vi "InitVI UI.vi"() -> ()   [LabVIEW 2015, in "Initialization.lvclass"]
uses:
  Initialization.lvclass
  <vilib>/NI/Configuration Framework/Node/NodeRef.ctl
  <vilib>/NI/Configuration Framework/Node/NISE_CEF_Node.lvclass
  <vilib>/NI/AMC/Message Queue.ctl
  <vilib>/NI/AMC/Message.ctl
  <vilib>/NI/Tools/Keyed Array/KeyedArray.ctl
  <vilib>/NI/Configuration Framework/Node/UserEventRef.ctl
  <vilib>/NI/Configuration Framework/Controls/EventCluster.ctl
  XML Controls/Execution Types.ctl
  Initialization.lvclass/Initialization.ctl
  Read Initialization VI Properties.vi
  Write Initialization VI Properties.vi
  <vilib>/NI/AMC/Create Single Message.vi
  <vilib>/NI/AMC/Update Message Routing Info.vi
  <vilib>/NI/AMC/Send Message.vi
  <vilib>/NI/AMC/AMC.lvlib
  Configuration Tool.lvlib
  <vilib>/NI/Tools/Keyed Array/Tools_KeyedArray.lvlib
  <vilib>/NI/Configuration Framework/NISE_CEF_TreeControl.lvlib
  VeriStand Custom Device XML Parser.lvlib
panel:
  in  "Main UI Tab":enum32{"Initialization VI"}(tab)
  in  "Show Documentation":bool
  in  "Execution":T1
  in  "Type":enum16{"Action", "VI"}(ring)
  in  "Position":enum16{"centered", "mouse pointer"}(ring)
  in  "Host Path to Initialization VI":path
  in  "user event":T2
  in  "main queue":T3
  in  "node ref":T4
  # "Dialog Settings"
  # "Dialog Settings"
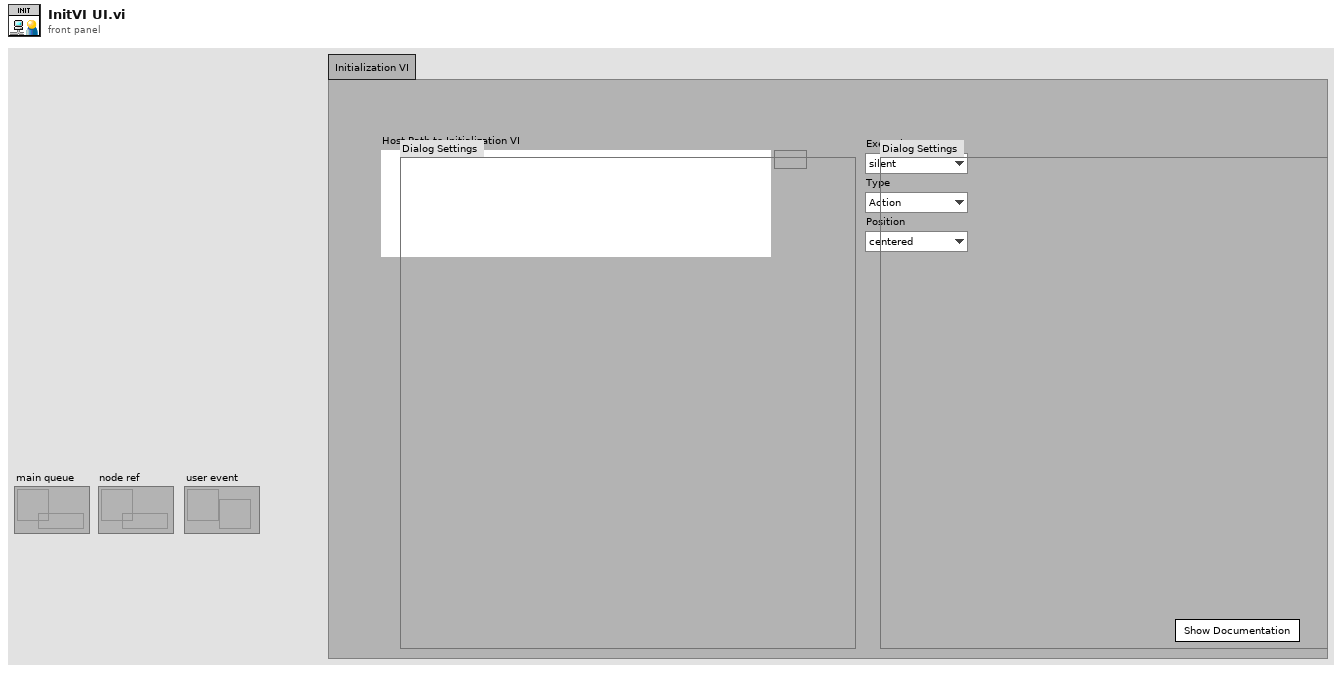
[diagram p1: front panel]
types:
  T1 = typedef "VeriStand Custom Device XML Parser.lvlib/Execution Types.ctl" = enum16{"silent", "modal", "floating", "default"}
  T2 = typedef "NISE_CEF_Node.lvclass/UserEventRef.ctl" = refnum<user-event>
  T3 = typedef "AMC.lvlib/Message Queue.ctl" = refnum<queue>
  T4 = typedef "NISE_CEF_Node.lvclass/NodeRef.ctl" = refnum<data-value>
  T5 = typedef "Initialization VI Properties.ctl" = cluster{"Execution":T6, "Path":T7, "Type":enum16{"Action", "VI"}, "Position":enum16{"centered", "mouse pointer"}}
  T6 = typedef "Execution Types.ctl" = enum16{"silent", "modal", "floating", "default"}
  T7 = typedef "Path Cluster.ctl" = cluster{"Path":path, "Path Type":enum16{"Absolute", "To Base", "To Common Doc Dir", "To Application Data Dir"}}
  T8 = enum16{"Absolute", "To Base", "To Common Doc Dir", "To Application Data Dir"}
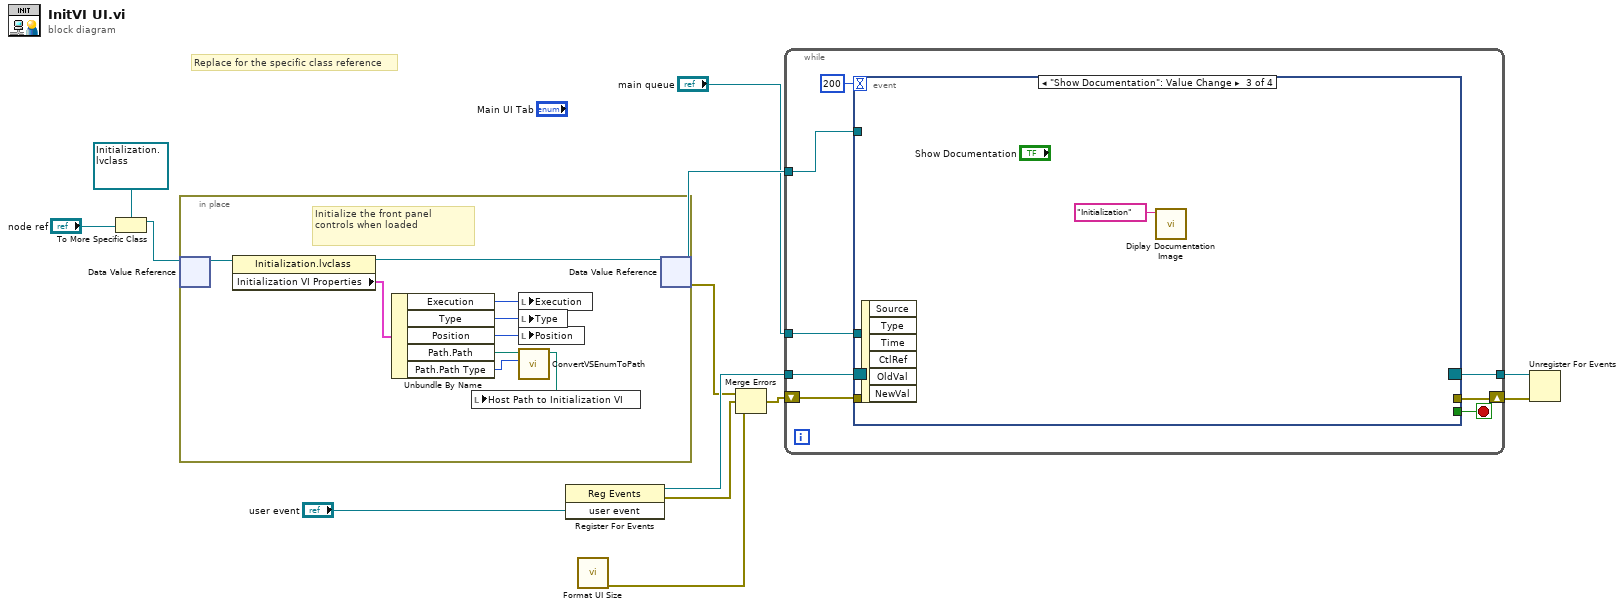
[diagram p0: block diagram]
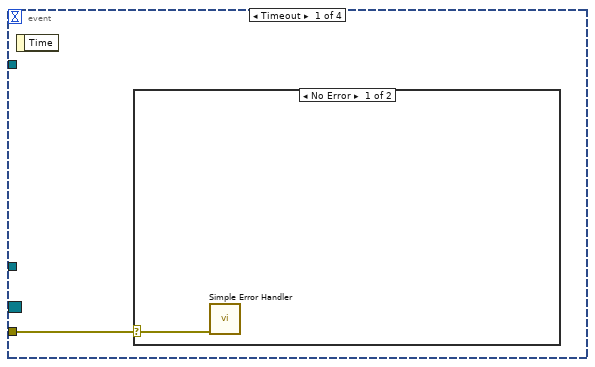
[diagram p2: hidden frame]
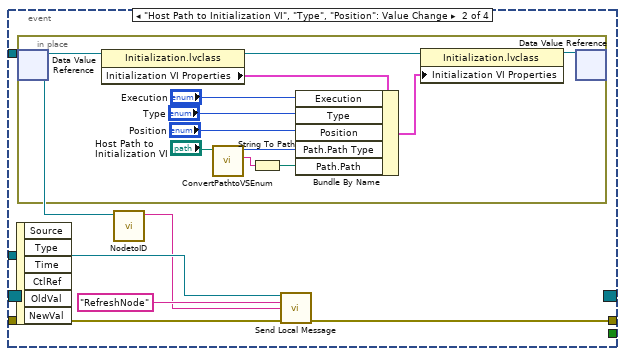
[diagram p4: hidden frame]
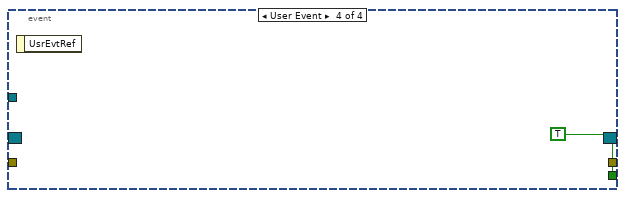
[diagram p5: hidden frame]
diagram:
  # "Replace for the specific class reference"
  n1 = To More Specific Class(target class=refnum<data-value> refnum ("data value reference"), reference="node ref") -> (specific class reference=w6:refnum<data-value>)  [unwired: 1 in, 1 out]
  n2 = in-place {
    # "Initialize the front panel controls when loaded"
    n3 = in-place-dvr #1(w6) -> (w22:refnum<class "Initialization.lvclass">)  [unwired: 1 out]
    n4 = property class="Initialization.lvclass"(reference=w22) -> (reference out=w21:refnum<class "Initialization.lvclass">, "Initialization VI Properties"=w20:T5)  [unwired: 1 in, 1 out]
    n5 = Unbundle By Name(w20) -> ("Execution"=w19:T6, "Type"=w18:enum16{"Action", "VI"}, "Position"=w17:enum16{"centered", "mouse pointer"}, "Path.Path"=w16:path, "Path.Path Type"=w15:T8)
    n6 = local write "Execution"(w19) -> ()
    n7 = local write "Type"(w18) -> ()
    n8 = local write "Position"(w17) -> ()
    n9 = call "ConvertVSEnumToPath.vi"("Source.Path Type"=w15, "Path In"=w16) -> ("appended path"=w14:path)  [unwired: 9 in]
    n10 = local write "Host Path to Initialization VI"(w14) -> ()
    n11 = in-place-dvr #1(w21) -> (w13:refnum<data-value>, w3:errorcluster)
  }
  n12 = register-events("user event") -> (reference out=w10:refnum<event-registration>, error out=w4:errorcluster)  [unwired: 2 in]
  n13 = call "Format UI Size.vi"() -> ("error out"=w1:errorcluster)  [unwired: 11 in]
  n14 = Merge Errors(w3, w4, w1) -> (w2:errorcluster)
  n15 = while {
    tunnel: w13 -> [w30]
    tunnel: "main queue" -> [w29]
    tunnel: w10 -> [w27]
    tunnel: [w26] -> w9
    shift-right: [w24] -> w8
    shift-left: w2 -> [w23]
    stop <- w25 stop-if-true
    n16 = event shown="[2] \"Show Documentation\": Value Change" {
      selector: w27 -> [_ _ _ _]
      dyn-events: [_ _ _ _] -> w26
      timeout: 200 -> [_ _ _ _]
      tunnel: w30 -> [_ w36 _ _]
      tunnel: w29 -> [_ w37 _ _]
      tunnel: [_ _ _ TRUE] -> w25
      tunnel: [_ w34 _ _] -> w24
      tunnel: w23 -> [w31 w33 _ _]
      event Timeout {
        n17 = event-data() -> ()  [unwired: 1 in, 1 out]
        n18 = case shown="No Error" w31 {
          selector: w31 -> [w32 _]
          frame No Error {
            n19 = call <vilib>:"Simple Error Handler.vi"("error in (no error)"=w32) -> ()  [unwired: 4 in, 5 out]
          }
          frame Error {
          }
        }
      }
      event "Host Path to Initialization VI", "Type", "Position": Value Change {
        n20 = event-data() -> ()  [unwired: 1 in, 6 out]
        n21 = in-place {
          n22 = in-place-dvr #2(w36) -> (w49:refnum<class "Initialization.lvclass">)  [unwired: 1 out]
          n23 = property class="Initialization.lvclass"(reference=w49) -> (reference out=w39:refnum<class "Initialization.lvclass">, "Initialization VI Properties"=w48:T5)  [unwired: 1 in, 1 out]
          n24 = call "ConvertPathtoVSEnum.vi"("Path In"="Host Path to Initialization VI") -> ("Remaining Path"=w47:string, "VS Enum Out"=w45:T8)  [unwired: 9 in]
          n25 = String To Path(string=w47) -> (path=w46:path)
          n26 = Bundle By Name(cluster=w48, "Execution"="Execution", "Type"="Type", "Position"="Position", "Path.Path Type"=w45, "Path.Path"=w46) -> (w40:T5)
          n27 = property class="Initialization.lvclass"(reference=w39, "Initialization VI Properties"=w40) -> (reference out=w50:refnum<class "Initialization.lvclass">)  [unwired: 1 in, 1 out]
          n28 = in-place-dvr #2(w50) -> ()  [unwired: 2 out]
        }
        n29 = call <vilib>:"NodetoID.vi"("node ref"=w36) -> ("ID"=w35:string)  [unwired: 9 in, 1 out]
        n30 = call <vilib>:"Send Local Message.vi"("message queue in"=w37, "message name"="RefreshNode" ("Message Name"), "message value"=w35, "error in"=w33) -> ("error out"=w34:errorcluster)  [unwired: 9 in, 2 out]
      }
      event "Show Documentation": Value Change {
        n31 = event-data() -> ()  [unwired: 1 in, 6 out]
        n32 = call "Diplay Documentation Image.vi"("Image Name"="Initialization") -> ()  [unwired: 10 in, 1 out]
      }
      event User Event {
        n33 = event-data() -> ()  [unwired: 1 in, 1 out]
      }
    }
  }
  n34 = Unregister For Events(event registration refnum=w9, error in=w8) -> ()  [unwired: 1 out]
